vi "test.vi"() -> ()   [LabVIEW 2017]
panel:
  out "x+y":timestamp
  out "output 3":dbl
  out "output 2":i32
  out "error out":errorcluster
  out "remaining string":string
  out "output 1":timestamp
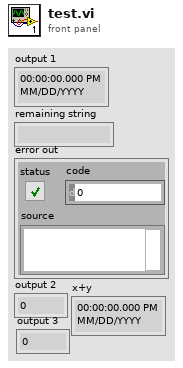
[diagram p1: front panel]
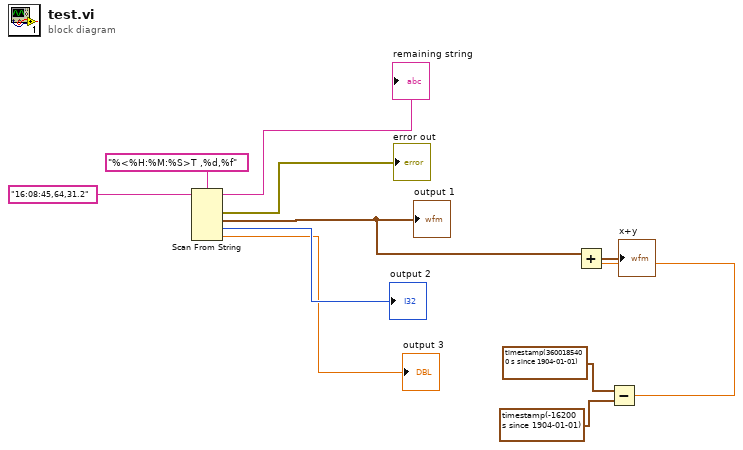
[diagram p0: block diagram]
diagram:
  n1 = Scan From String(format string="%<%H:%M:%S>T ,%d,%f", input string="16:08:45,64,31.2") -> (remaining string=→"remaining string":string, error out=→"error out":errorcluster, output 1=w5:timestamp, output 2=→"output 2":i32, output 3=→"output 3":dbl)  [unwired: 5 in, 1 out]
  "output 1" <- w5
  n2 = Subtract(x=timestamp(3600185400 s since 1904-01-01), y=timestamp(-16200 s since 1904-01-01)) -> (x-y=w1:dbl)
  n3 = Add(x=w5, y=w1) -> (x+y=→"x+y":timestamp)
